vi "working pid.vi"() -> ()   [LabVIEW 2018]
uses:
  <vilib>/DAQmx/write.llb/DAQmx Write (Digital 1D Bool 1Chan 1Samp).vi
  <vilib>/DAQmx/create/channels.llb/DAQmx Create Channel (DO-Digital Output).vi
  <vilib>/addons/control/pid/pid.llb/PID (DBL).vi
  <vilib>/DAQmx/miscellaneous.llb/DAQmx Fill In Error Info.vi
  <vilib>/addons/control/pid/NI_PID_pid.lvlib
  <vilib>/ptbypt/NI_PtbyPt.lvlib
panel:
  out "Actual Pressure in the muscle 12":dbl(knob) scale=0.0..40.0
  out "Actual Pressure in the muscle 11":dbl(knob) scale=0.0..40.0
  out "Actual Pressure in the muscle 6":dbl(knob) scale=0.0..30.0
  out "Actual Pressure in the muscle 7":dbl(knob) scale=0.0..30.0
  out "Actual Pressure in the muscle 2":dbl(knob) scale=0.0..30.0
  out "Actual Pressure in the muscle 4":dbl(knob) scale=0.0..30.0
  out "Actual Pressure in the muscle 1":dbl(knob) scale=0.0..30.0
  in  "stop (F) 4":bool caption="stop (F)"
  out "Waveform Chart 2":dbl[][](graph)
  in  "PID gains 2":T1={"proportional gain (Kc)"=0.001, "integral time (Ti, min)"=30.0, "derivative time (Td, min)"=0.0} {"derivative time (Td, min)" format="%.3f"; "integral time (Ti, min)" format="%.3f"; "proportional gain (Kc)" format="%.3f"}
  out "PWM Output 2":bool
  in  "stop 2":bool
  in  "Pressure Setpoint 2":dbl=500.0 format="%.2f"
  in  "Pressure Setpoint":dbl=500.0 format="%.2f"
  in  "stop":bool
  out "PWM Output":bool
  in  "PID gains":T1={"proportional gain (Kc)"=0.001, "integral time (Ti, min)"=30.0, "derivative time (Td, min)"=0.0} {"derivative time (Td, min)" format="%.3f"; "integral time (Ti, min)" format="%.3f"; "proportional gain (Kc)" format="%.3f"}
  out "Waveform Chart":dbl[][](graph)
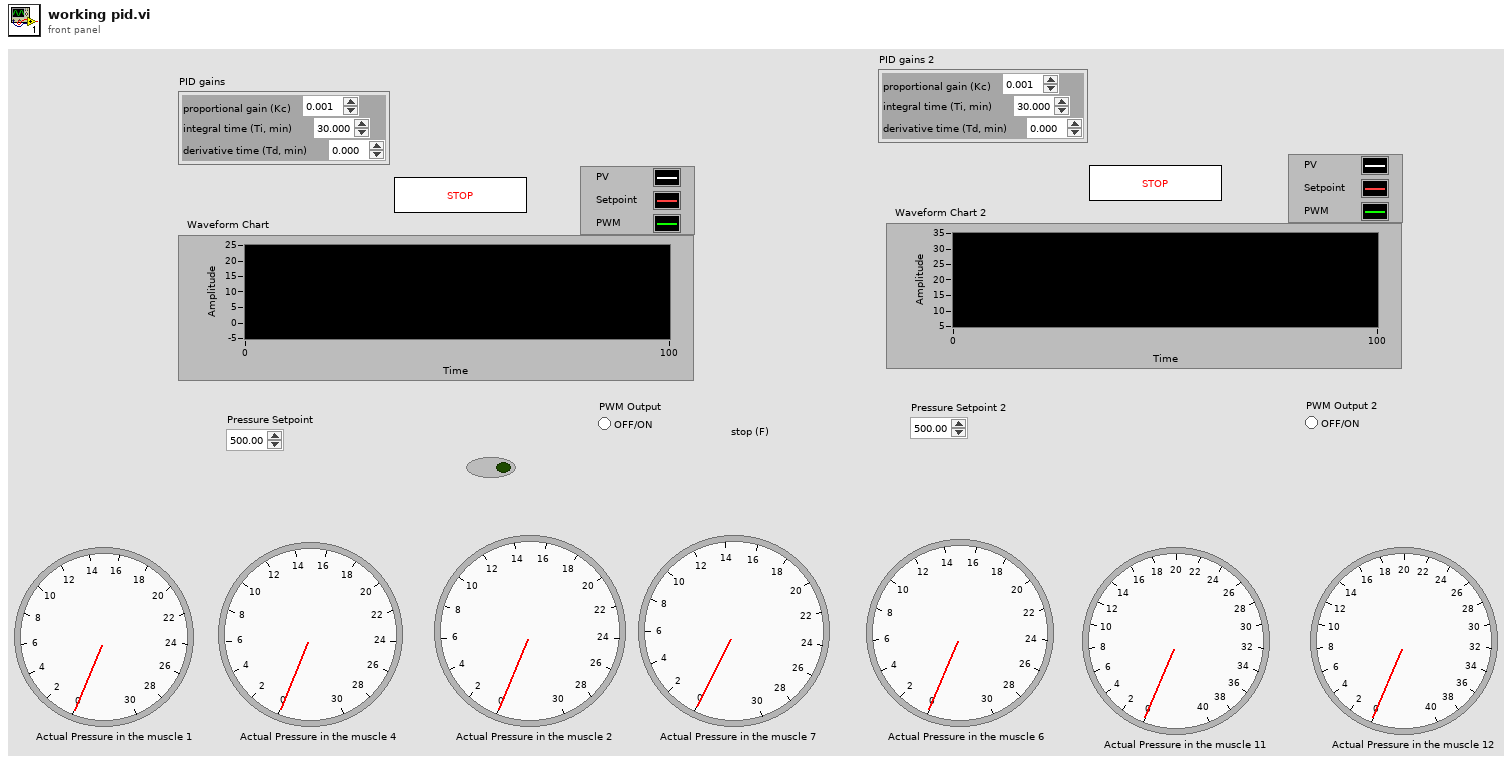
[diagram p1: front panel]
types:
  T1 = cluster{"proportional gain (Kc)":dbl, "integral time (Ti, min)":dbl, "derivative time (Td, min)":dbl}
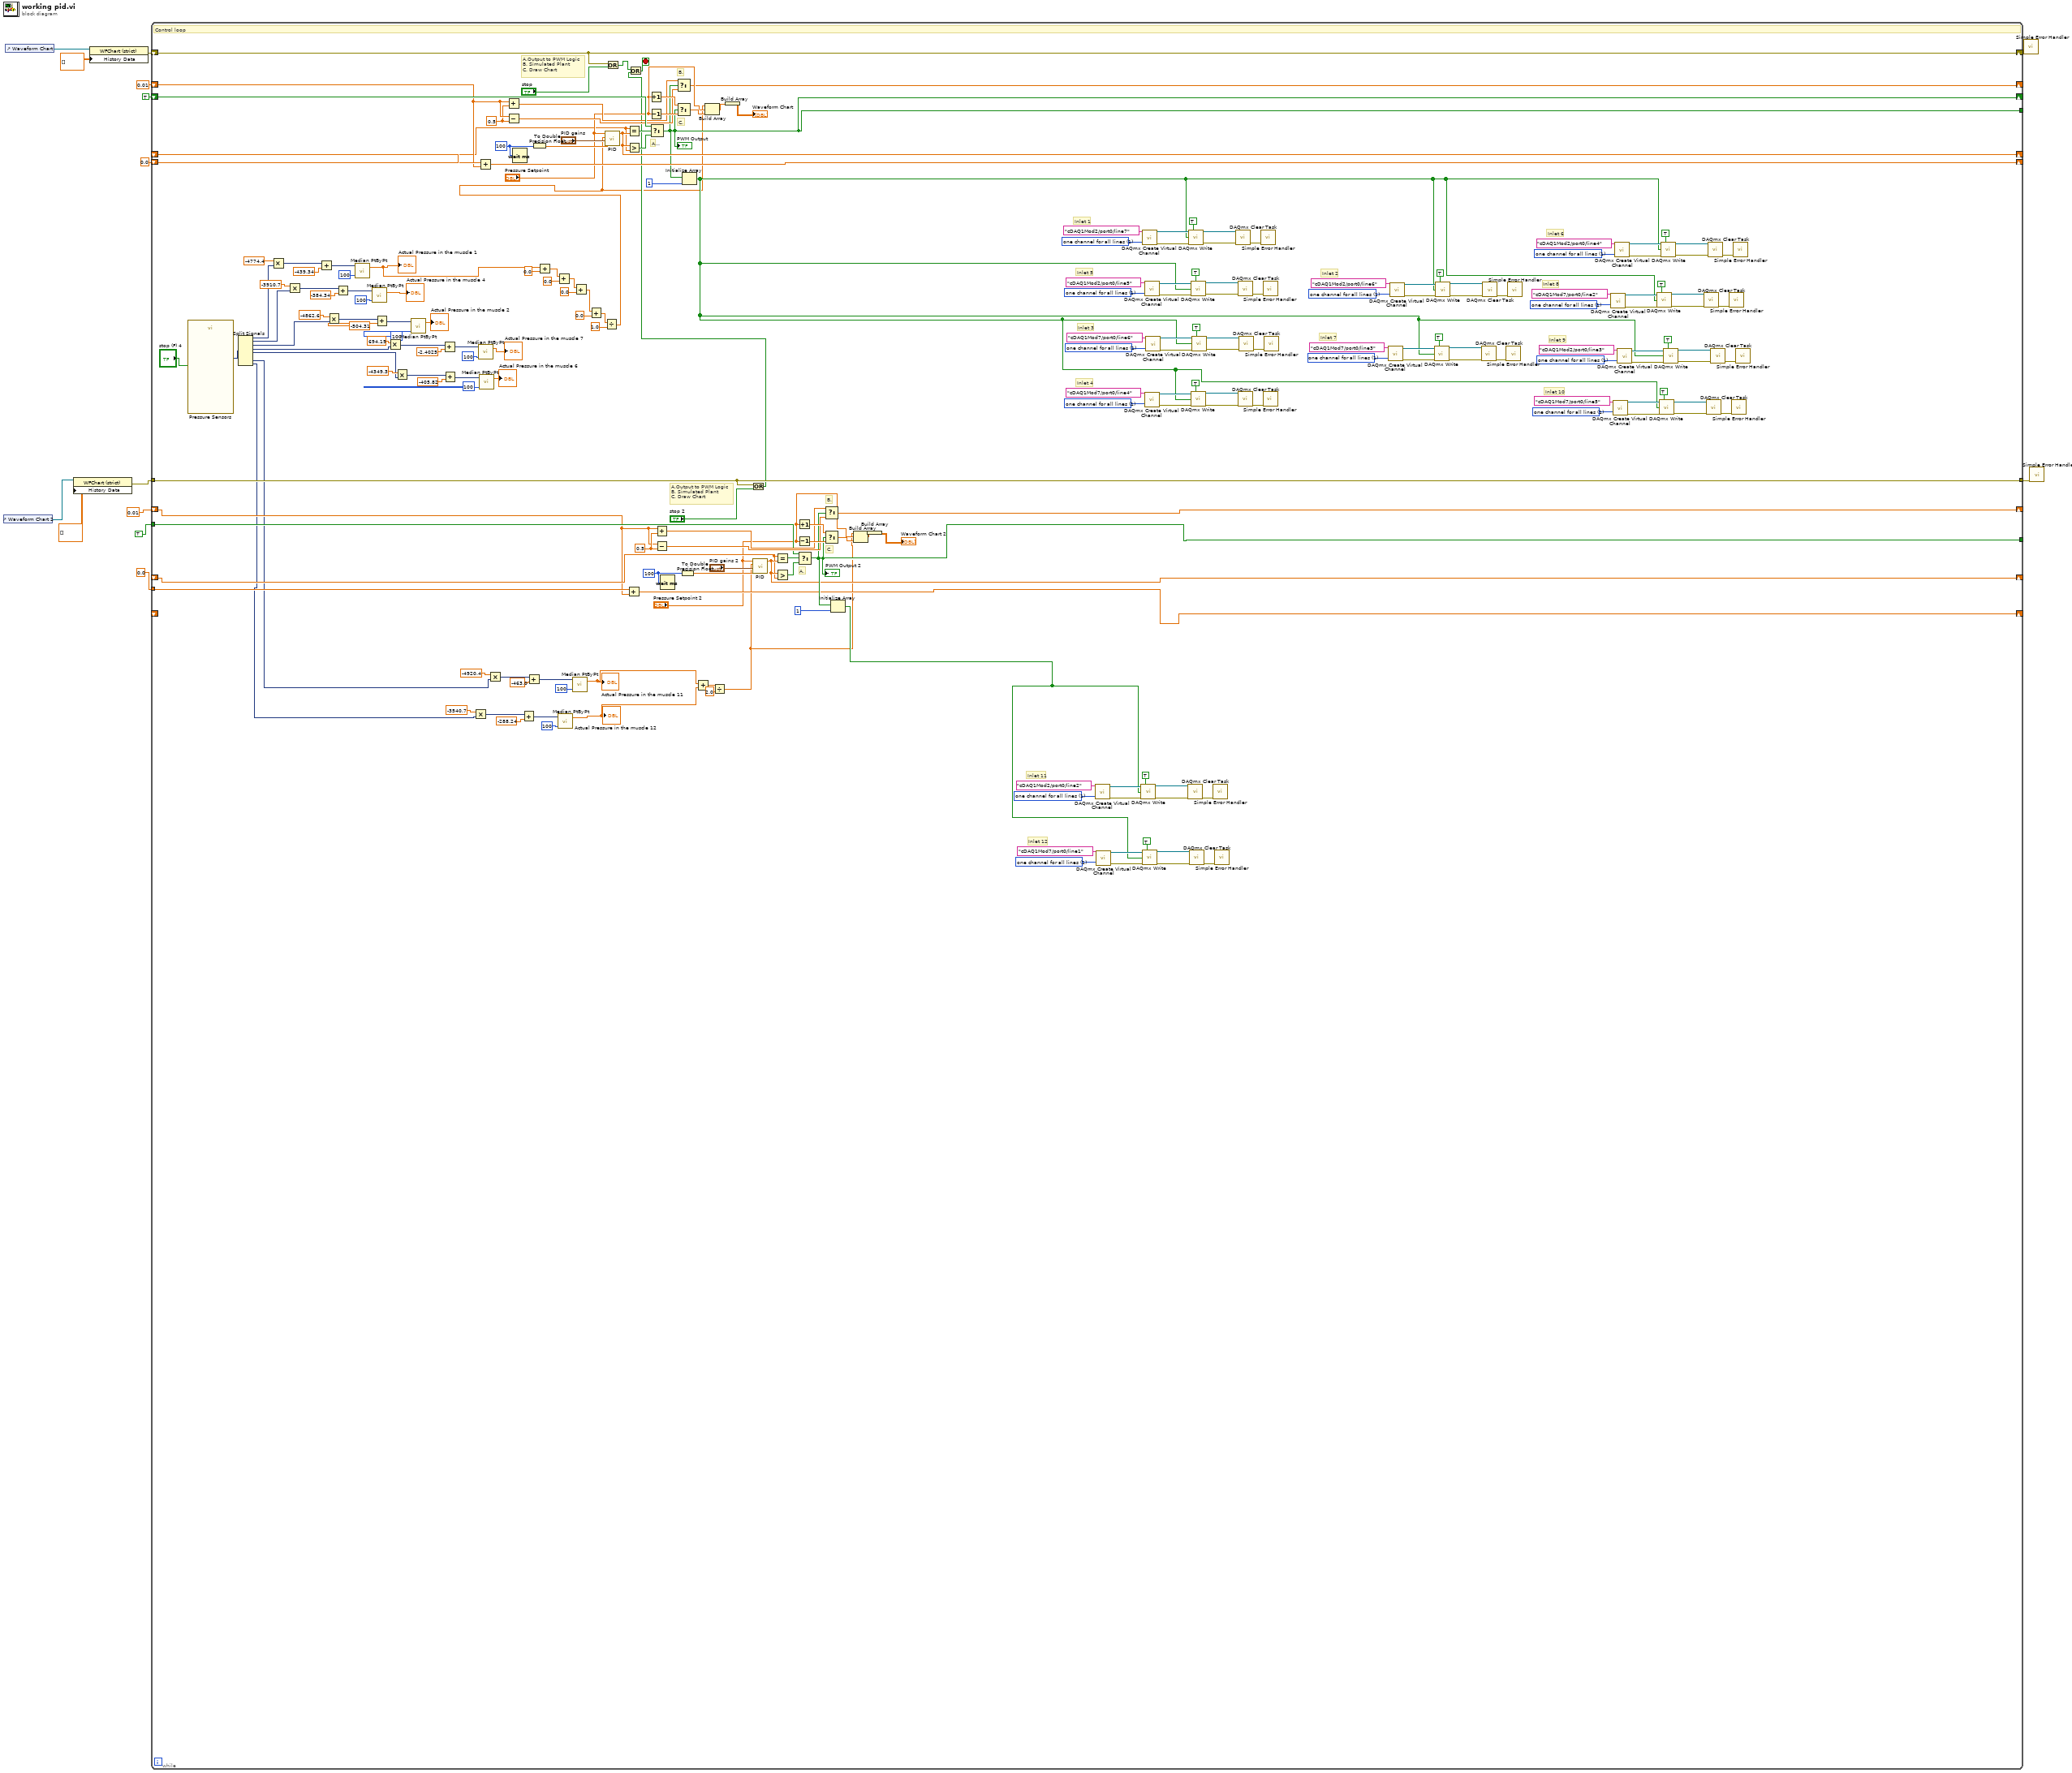
[diagram p0: block diagram]
diagram:
  w13 = 0.0 ("output")
  n1 = control-ref of="Waveform Chart 2"() -> (w7:refnum<vi>)
  n2 = control-ref of="Waveform Chart"() -> (w11:refnum<vi>)
  n3 = property class="WFChart (strict)"(reference=w7, "History Data"=dbl[][] []) -> (error out=w5:errorcluster)  [unwired: 1 in, 1 out]
  n4 = property class="WFChart (strict)"(reference=w11, "History Data"=dbl[][] []) -> (error out=w10:errorcluster)  [unwired: 1 in, 1 out]
  n5 = while {
    shift-right: [w226] -> _
    shift-left: w13 -> [w190]
    shift-right: [w210] -> _
    shift-left: TRUE -> [w225]
    shift-right: [w223] -> _
    shift-left: w13 -> [w224]
    shift-right: [w187] -> _
    shift-left: 0.01 -> [w222]
    shift-right: [w221] -> w9
    shift-left: w10 -> [w221]
    tunnel: [w210] -> _
    tunnel: w5 -> [w188]
    tunnel: TRUE -> [w191]
    tunnel: 0.0 ("output") -> [w189]
    tunnel: [w188] -> w2
    shift-right: [w186] -> _
    shift-left: 0.01 -> [w179]
    tunnel: [w185] -> _
    shift-right: [w184] -> _
    shift-left: _ -> [w183]
    shift-right: [w178] -> _
    shift-left: _ -> [_]
    stop <- w181 stop-if-true
    w82 = 1 items=["one channel for each line", "one channel for all lines"] ("line grouping")
    w90 = 1 items=["one channel for each line", "one channel for all lines"] ("line grouping")
    w99 = 1 items=["one channel for each line", "one channel for all lines"] ("line grouping")
    w107 = 1 items=["one channel for each line", "one channel for all lines"] ("line grouping")
    w115 = 1 items=["one channel for each line", "one channel for all lines"] ("line grouping")
    w123 = 1 items=["one channel for each line", "one channel for all lines"] ("line grouping")
    w131 = 1 items=["one channel for each line", "one channel for all lines"] ("line grouping")
    w139 = 1 items=["one channel for each line", "one channel for all lines"] ("line grouping")
    w147 = 1 items=["one channel for each line", "one channel for all lines"] ("line grouping")
    w155 = 1 items=["one channel for each line", "one channel for all lines"] ("line grouping")
    w163 = 1 items=["one channel for each line", "one channel for all lines"] ("line grouping")
    w171 = 1 items=["one channel for each line", "one channel for all lines"] ("line grouping")
    w196 = 0.5 ("x")
    w204 = u32 100 ("milliseconds to wait")
    w213 = 0.5 ("x")
    w227 = u32 100 ("milliseconds to wait")
    # "Inlet 12"
    # "Inlet 11"
    # "Inlet 10"
    # "Inlet 9"
    # "Inlet 8"
    # "Inlet 6"
    # "Inlet 7"
    # "Inlet 2"
    # "Inlet 4"
    # "Inlet 3"
    # "Inlet 5"
    # "Inlet 1"
    # "B."
    # "C."
    # "A."
    # "A.Output to PWM Logic \nB. Simulated Plant\nC. Draw Chart"
    # "B."
    # "C."
    # "A."
    # "A.Output to PWM Logic \nB. Simulated Plant\nC. Draw Chart"
    # "Control loop"
    n6 = call "Pressure Sensors"("stop (T)"="stop (F) 4") -> ("data"=w77:dynamicdata)  [unwired: 16 in, 2 out]
    n7 = Split Signals(w77) -> (w76:dynamicdata, w66:dynamicdata, w60:dynamicdata, w54:dynamicdata, w48:dynamicdata, w42:dynamicdata, w36:dynamicdata)  [unwired: 8 in, 1 out]
    n8 = Multiply(x=-4774.4, y=w76) -> (x*y=w79:dynamicdata)
    n9 = Multiply(x=-3910.7, y=w66) -> (x*y=w71:dynamicdata)
    n10 = Add(x=w79, y=-439.34) -> (x+y=w73:dynamicdata)
    n11 = Multiply(x=-4862.6, y=w60) -> (x*y=w65:dynamicdata)
    n12 = Add(x=w71, y=-384.34) -> (x+y=w68:dynamicdata)
    n13 = call <vilib>:"Median PtByPt.vi"("sample length"=100, "x"=w73) -> ("median"=w35:dbl)  [unwired: 2 in, 1 out]
    "Actual Pressure in the muscle 1" <- w35
    n14 = call <vilib>:"Median PtByPt.vi"("sample length"=100, "x"=w68) -> ("median"=→"Actual Pressure in the muscle 4":dbl)  [unwired: 2 in, 1 out]
    n15 = Add(x=w65, y=-504.31) -> (x+y=w62:dynamicdata)
    n16 = Multiply(x=694.19, y=w54) -> (x*y=w59:dynamicdata)
    n17 = Multiply(x=-4349.3, y=w48) -> (x*y=w53:dynamicdata)
    n18 = call <vilib>:"Median PtByPt.vi"("sample length"=100, "x"=w62) -> ("median"=→"Actual Pressure in the muscle 2":dbl)  [unwired: 2 in, 1 out]
    n19 = Add(x=w59, y=-2.4025) -> (x+y=w56:dynamicdata)
    n20 = Add(x=w53, y=-405.82) -> (x+y=w50:dynamicdata)
    n21 = Multiply(x=-3540.7, y=w36) -> (x*y=w41:dynamicdata)
    n22 = Add(x=w224, y=w222) -> (x+y=w223:dbl)
    n23 = call <vilib>:"Median PtByPt.vi"("sample length"=100, "x"=w56) -> ("median"=→"Actual Pressure in the muscle 7":dbl)  [unwired: 2 in, 1 out]
    n24 = call <vilib>:"Median PtByPt.vi"("sample length"=100, "x"=w50) -> ("median"=→"Actual Pressure in the muscle 6":dbl)  [unwired: 2 in, 1 out]
    n25 = Multiply(x=-4920.4, y=w42) -> (x*y=w47:dynamicdata)
    n26 = Add(x=w222, y=w213) -> (x+y=w214:dbl)
    n27 = Subtract(x=w222, y=w213) -> (x-y=w212:dbl)
    n28 = Wait (ms)(milliseconds to wait=w227) -> ()  [unwired: 1 out]
    n29 = Add(x=w41, y=-288.24) -> (x+y=w38:dynamicdata)
    n30 = Add(x=w47, y=-463.0) -> (x+y=w44:dynamicdata)
    n31 = To Double Precision Float(number=w227) -> (double precision float=w211:dbl)
    n32 = Add(x=w35, y=0.0) -> (x+y=w33:dbl)
    n33 = Add(x=w33, y=0.0) -> (x+y=w31:dbl)
    n34 = call <vilib>:"Median PtByPt.vi"("sample length"=100, "x"=w38) -> ("median"=w24:dbl)  [unwired: 2 in, 1 out]
    "Actual Pressure in the muscle 12" <- w24
    n35 = call <vilib>:"Median PtByPt.vi"("sample length"=100, "x"=w44) -> ("median"=w25:dbl)  [unwired: 2 in, 1 out]
    "Actual Pressure in the muscle 11" <- w25
    n36 = Add(x=w31, y=0.0) -> (x+y=w29:dbl)
    n37 = Add(x=w29, y=0.0) -> (x+y=w27:dbl)
    n38 = Divide(x=w27, y=1.0) -> (x/y=w17:dbl)
    n39 = call-poly <vilib>:"PID.vi"("dt (s)"=w211, "PID gains"="PID gains", "process variable"=w17, "setpoint"="Pressure Setpoint") -> ("output"=w226:dbl)  [unwired: 6 in, 1 out]
    n40 = Or(x=w221, y="stop") -> (x .or. y?=w182:bool)
    n41 = Add(x=w189, y=w179) -> (x+y=w178:dbl)
    n42 = Equal?(x=w190, y=w226) -> (x = y?=w220:bool)
    n43 = Greater?(x=w226, y=w190) -> (0:w219:bool)
    n44 = Increment(x="Pressure Setpoint") -> (x+1=w218:dbl)
    n45 = Decrement(x="Pressure Setpoint") -> (x-1=w217:dbl)
    n46 = Select(t=w225, s=w220, f=w219) -> (s? t:f=w210:bool)
    "PWM Output" <- w210
    n47 = Add(x=w179, y=w196) -> (x+y=w197:dbl)
    n48 = Subtract(x=w179, y=w196) -> (x-y=w195:dbl)
    n49 = Wait (ms)(milliseconds to wait=w204) -> ()  [unwired: 1 out]
    n50 = Select(t=w214, s=w210, f=w212) -> (s? t:f=w187:dbl)
    n51 = Select(t=w218, s=w210, f=w217) -> (s? t:f=w216:dbl)
    n52 = To Double Precision Float(number=w204) -> (double precision float=w194:dbl)
    n53 = Initialize Array(w210, 1 ("dimension size")) -> (w97:bool[])
    n54 = Add(x=w25, y=w24) -> (x+y=w23:dbl)
    n55 = Build Array(w17, "Pressure Setpoint", w216) -> (w215:dbl[])
    n56 = Divide(x=w23, y=2.0) -> (x/y=w15:dbl)
    n57 = Build Array(w215) -> (→"Waveform Chart":dbl[][])
    n58 = Or(x=w188, y="stop 2") -> (x .or. y?=w180:bool)
    n59 = Or(x=w182, y=w180) -> (x .or. y?=w181:bool)
    n60 = call-poly <vilib>:"PID.vi"("dt (s)"=w194, "PID gains"="PID gains 2", "process variable"=w15, "setpoint"="Pressure Setpoint 2") -> ("output"=w184:dbl)  [unwired: 6 in, 1 out]
    n61 = Equal?(x=w183, y=w184) -> (x = y?=w203:bool)
    n62 = Greater?(x=w184, y=w183) -> (0:w202:bool)
    n63 = Increment(x="Pressure Setpoint 2") -> (x+1=w201:dbl)
    n64 = Decrement(x="Pressure Setpoint 2") -> (x-1=w200:dbl)
    n65 = Select(t=w191, s=w203, f=w202) -> (s? t:f=w185:bool)
    "PWM Output 2" <- w185
    n66 = Select(t=w197, s=w185, f=w195) -> (s? t:f=w186:dbl)
    n67 = Select(t=w201, s=w185, f=w200) -> (s? t:f=w199:dbl)
    n68 = Initialize Array(w185, 1 ("dimension size")) -> (w80:bool[])
    n69 = Build Array(w15, "Pressure Setpoint 2", w199) -> (w198:dbl[])
    n70 = Build Array(w198) -> (→"Waveform Chart 2":dbl[][])
    n71 = call-poly <vilib>:"DAQmx Create Virtual Channel.vi"("lines"=tag "cDAQ1Mod2/port0/line2", "line grouping"=w90) -> ("task out"=w92:refnum<k21>, "error out"=w91:errorcluster)  [unwired: 12 in]
    n72 = call-poly <vilib>:"DAQmx Create Virtual Channel.vi"("lines"=tag "cDAQ1Mod7/port0/line1", "line grouping"=w82) -> ("task out"=w84:refnum<k21>, "error out"=w83:errorcluster)  [unwired: 12 in]
    n73 = call-poly <vilib>:"DAQmx Write.vi"("task/channels in"=w92, "auto start"=TRUE, "data"=w80, "error in"=w91) -> ("task out"=w94:refnum<k21>, "error out"=w95:errorcluster)  [unwired: 9 in, 1 out]
    n74 = call-poly <vilib>:"DAQmx Create Virtual Channel.vi"("lines"=tag "cDAQ1Mod2/port0/line7", "line grouping"=w171) -> ("task out"=w173:refnum<k21>, "error out"=w172:errorcluster)  [unwired: 12 in]
    n75 = call-poly <vilib>:"DAQmx Write.vi"("task/channels in"=w84, "auto start"=TRUE, "data"=w80, "error in"=w83) -> ("task out"=w86:refnum<k21>, "error out"=w87:errorcluster)  [unwired: 9 in, 1 out]
    n76 = call-poly <vilib>:"DAQmx Create Virtual Channel.vi"("lines"=tag "cDAQ1Mod2/port0/line5", "line grouping"=w163) -> ("task out"=w165:refnum<k21>, "error out"=w164:errorcluster)  [unwired: 12 in]
    n77 = call-poly <vilib>:"DAQmx Create Virtual Channel.vi"("lines"=tag "cDAQ1Mod7/port0/line4", "line grouping"=w147) -> ("task out"=w149:refnum<k21>, "error out"=w148:errorcluster)  [unwired: 12 in]
    n78 = call-poly <vilib>:"DAQmx Create Virtual Channel.vi"("lines"=tag "cDAQ1Mod7/port0/line6", "line grouping"=w155) -> ("task out"=w157:refnum<k21>, "error out"=w156:errorcluster)  [unwired: 12 in]
    n79 = call <vilib>:"DAQmx Clear Task.vi"("task in"=w94, "error in"=w95) -> ("error out"=w89:errorcluster)  [unwired: 13 in]
    n80 = call-poly <vilib>:"DAQmx Write.vi"("task/channels in"=w173, "auto start"=TRUE, "data"=w97, "error in"=w172) -> ("task out"=w175:refnum<k21>, "error out"=w176:errorcluster)  [unwired: 9 in, 1 out]
    n81 = call <vilib>:"DAQmx Clear Task.vi"("task in"=w86, "error in"=w87) -> ("error out"=w81:errorcluster)  [unwired: 13 in]
    n82 = call-poly <vilib>:"DAQmx Write.vi"("task/channels in"=w165, "auto start"=TRUE, "data"=w97, "error in"=w164) -> ("task out"=w167:refnum<k21>, "error out"=w168:errorcluster)  [unwired: 9 in, 1 out]
    n83 = call-poly <vilib>:"DAQmx Write.vi"("task/channels in"=w149, "auto start"=TRUE, "data"=w97, "error in"=w148) -> ("task out"=w151:refnum<k21>, "error out"=w152:errorcluster)  [unwired: 9 in, 1 out]
    n84 = call-poly <vilib>:"DAQmx Write.vi"("task/channels in"=w157, "auto start"=TRUE, "data"=w97, "error in"=w156) -> ("task out"=w159:refnum<k21>, "error out"=w160:errorcluster)  [unwired: 9 in, 1 out]
    n85 = call <vilib>:"Simple Error Handler.vi"("error in (no error)"=w89) -> ()  [unwired: 4 in, 5 out]
    n86 = call <vilib>:"Simple Error Handler.vi"("error in (no error)"=w81) -> ()  [unwired: 4 in, 5 out]
    n87 = call <vilib>:"DAQmx Clear Task.vi"("task in"=w175, "error in"=w176) -> ("error out"=w170:errorcluster)  [unwired: 13 in]
    n88 = call <vilib>:"DAQmx Clear Task.vi"("task in"=w167, "error in"=w168) -> ("error out"=w162:errorcluster)  [unwired: 13 in]
    n89 = call <vilib>:"DAQmx Clear Task.vi"("task in"=w151, "error in"=w152) -> ("error out"=w146:errorcluster)  [unwired: 13 in]
    n90 = call <vilib>:"DAQmx Clear Task.vi"("task in"=w159, "error in"=w160) -> ("error out"=w154:errorcluster)  [unwired: 13 in]
    n91 = call <vilib>:"Simple Error Handler.vi"("error in (no error)"=w170) -> ()  [unwired: 4 in, 5 out]
    n92 = call <vilib>:"Simple Error Handler.vi"("error in (no error)"=w162) -> ()  [unwired: 4 in, 5 out]
    n93 = call <vilib>:"Simple Error Handler.vi"("error in (no error)"=w146) -> ()  [unwired: 4 in, 5 out]
    n94 = call <vilib>:"Simple Error Handler.vi"("error in (no error)"=w154) -> ()  [unwired: 4 in, 5 out]
    n95 = call-poly <vilib>:"DAQmx Create Virtual Channel.vi"("lines"=tag "cDAQ1Mod7/port0/line3", "line grouping"=w131) -> ("task out"=w133:refnum<k21>, "error out"=w132:errorcluster)  [unwired: 12 in]
    n96 = call-poly <vilib>:"DAQmx Create Virtual Channel.vi"("lines"=tag "cDAQ1Mod2/port0/line6", "line grouping"=w139) -> ("task out"=w141:refnum<k21>, "error out"=w140:errorcluster)  [unwired: 12 in]
    n97 = call-poly <vilib>:"DAQmx Write.vi"("task/channels in"=w133, "auto start"=TRUE, "data"=w97, "error in"=w132) -> ("task out"=w135:refnum<k21>, "error out"=w136:errorcluster)  [unwired: 9 in, 1 out]
    n98 = call-poly <vilib>:"DAQmx Write.vi"("task/channels in"=w141, "auto start"=TRUE, "data"=w97, "error in"=w140) -> ("task out"=w143:refnum<k21>, "error out"=w144:errorcluster)  [unwired: 9 in, 1 out]
    n99 = call <vilib>:"DAQmx Clear Task.vi"("task in"=w135, "error in"=w136) -> ("error out"=w130:errorcluster)  [unwired: 13 in]
    n100 = call <vilib>:"DAQmx Clear Task.vi"("task in"=w143, "error in"=w144) -> ("error out"=w138:errorcluster)  [unwired: 13 in]
    n101 = call <vilib>:"Simple Error Handler.vi"("error in (no error)"=w130) -> ()  [unwired: 4 in, 5 out]
    n102 = call <vilib>:"Simple Error Handler.vi"("error in (no error)"=w138) -> ()  [unwired: 4 in, 5 out]
    n103 = call-poly <vilib>:"DAQmx Create Virtual Channel.vi"("lines"=tag "cDAQ1Mod7/port0/line2", "line grouping"=w115) -> ("task out"=w117:refnum<k21>, "error out"=w116:errorcluster)  [unwired: 12 in]
    n104 = call-poly <vilib>:"DAQmx Create Virtual Channel.vi"("lines"=tag "cDAQ1Mod7/port0/line5", "line grouping"=w99) -> ("task out"=w101:refnum<k21>, "error out"=w100:errorcluster)  [unwired: 12 in]
    n105 = call-poly <vilib>:"DAQmx Create Virtual Channel.vi"("lines"=tag "cDAQ1Mod2/port0/line4", "line grouping"=w123) -> ("task out"=w125:refnum<k21>, "error out"=w124:errorcluster)  [unwired: 12 in]
    n106 = call-poly <vilib>:"DAQmx Create Virtual Channel.vi"("lines"=tag "cDAQ1Mod2/port0/line3", "line grouping"=w107) -> ("task out"=w109:refnum<k21>, "error out"=w108:errorcluster)  [unwired: 12 in]
    n107 = call-poly <vilib>:"DAQmx Write.vi"("task/channels in"=w117, "auto start"=TRUE, "data"=w97, "error in"=w116) -> ("task out"=w119:refnum<k21>, "error out"=w120:errorcluster)  [unwired: 9 in, 1 out]
    n108 = call-poly <vilib>:"DAQmx Write.vi"("task/channels in"=w101, "auto start"=TRUE, "data"=w97, "error in"=w100) -> ("task out"=w103:refnum<k21>, "error out"=w104:errorcluster)  [unwired: 9 in, 1 out]
    n109 = call-poly <vilib>:"DAQmx Write.vi"("task/channels in"=w125, "auto start"=TRUE, "data"=w97, "error in"=w124) -> ("task out"=w127:refnum<k21>, "error out"=w128:errorcluster)  [unwired: 9 in, 1 out]
    n110 = call-poly <vilib>:"DAQmx Write.vi"("task/channels in"=w109, "auto start"=TRUE, "data"=w97, "error in"=w108) -> ("task out"=w111:refnum<k21>, "error out"=w112:errorcluster)  [unwired: 9 in, 1 out]
    n111 = call <vilib>:"DAQmx Clear Task.vi"("task in"=w119, "error in"=w120) -> ("error out"=w114:errorcluster)  [unwired: 13 in]
    n112 = call <vilib>:"DAQmx Clear Task.vi"("task in"=w103, "error in"=w104) -> ("error out"=w98:errorcluster)  [unwired: 13 in]
    n113 = call <vilib>:"DAQmx Clear Task.vi"("task in"=w127, "error in"=w128) -> ("error out"=w122:errorcluster)  [unwired: 13 in]
    n114 = call <vilib>:"DAQmx Clear Task.vi"("task in"=w111, "error in"=w112) -> ("error out"=w106:errorcluster)  [unwired: 13 in]
    n115 = call <vilib>:"Simple Error Handler.vi"("error in (no error)"=w114) -> ()  [unwired: 4 in, 5 out]
    n116 = call <vilib>:"Simple Error Handler.vi"("error in (no error)"=w98) -> ()  [unwired: 4 in, 5 out]
    n117 = call <vilib>:"Simple Error Handler.vi"("error in (no error)"=w122) -> ()  [unwired: 4 in, 5 out]
    n118 = call <vilib>:"Simple Error Handler.vi"("error in (no error)"=w106) -> ()  [unwired: 4 in, 5 out]
  }
  n119 = call <vilib>:"Simple Error Handler.vi"("error in (no error)"=w9) -> ()  [unwired: 4 in, 5 out]
  n120 = call <vilib>:"Simple Error Handler.vi"("error in (no error)"=w2) -> ()  [unwired: 4 in, 5 out]
